vi "Open Shutter.vi"(8 "error in (no error)":errorcluster, 10 "Open Shutter":bool, 11 "Topas4 in":refnum<class "Topas4.lvclass">) -> (0 "error out":errorcluster, 3 "Topas4 out":refnum<class "Topas4.lvclass">)   [LabVIEW 2020, in "Topas4.lvclass"]
uses:
  Topas4.lvclass
  Topas4.lvclass/Topas4.ctl
  Topas4-LabVIEW-Driver/Library/Topas4.lvlib
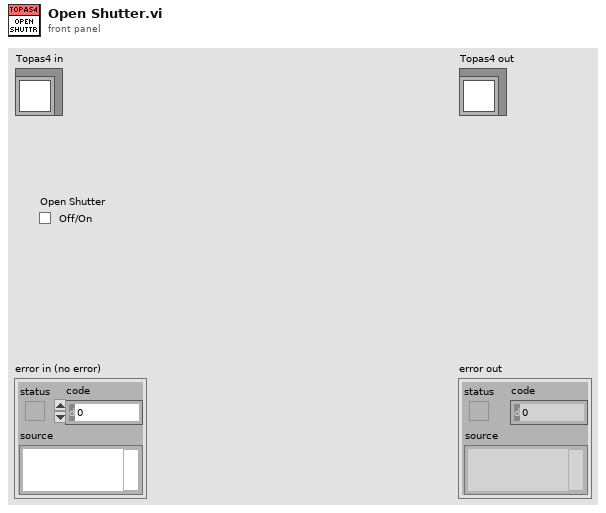
[diagram p1: front panel]
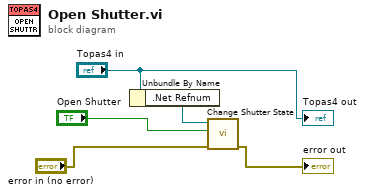
[diagram p0: block diagram]
diagram:
  n1 = Unbundle By Name("Topas4 in") -> (".Net Refnum"=w4:refnum<k24>)
  n2 = call "Change Shutter State.vi"("error in"="error in (no error)", "open"="Open Shutter", "reference"=w4) -> ("error out"=→"error out":errorcluster)  [unwired: 7 in, 1 out]
  "Topas4 out" <- "Topas4 in"
